vi "Disabled.vi"(7 "Robot Mode":T2, 10 "Match Info":T1={"Autonomous Elapsed Seconds"=0.0, "TeleOp Elapsed Seconds"=0.0, "Disabled Elapsed Seconds"=0.0, "Visited Autonomous"=FALSE, "Visited TeleOp"=FALSE, "Visited Disabled"=FALSE, "Autonomous Settings"={"Autonomous Style"=enum."Independent", "VI Refnum"=refnum}}, 11 "Call Context":T3) -> ()   [LabVIEW 2015]
doc: "This VI is called each time a disabled packet is received from the DS. It is often used to prepare for the next robot mode, to calibrate sensors, etc."
uses:
  <vilib>/Rock Robotics/WPI/DriverStation/WPI_DriverStationDerivedRobotMode.ctl
  <vilib>/Rock Robotics/WPI/DriverStation/WPI_DriverStationRobotMode2.ctl
  <vilib>/Rock Robotics/WPI/DriverStation/WPI_DriverStationMatch Info.ctl
  Robot Global Data.vi
panel:
  # "DISABLED.VI"
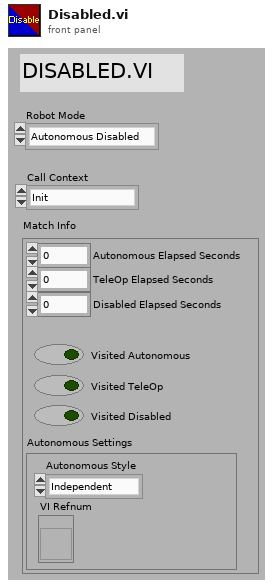
[diagram p1: front panel]
types:
  T1 = typedef "WPI_DriverStationMatch Info.ctl" = cluster{"Autonomous Elapsed Seconds":dbl, "TeleOp Elapsed Seconds":dbl, "Disabled Elapsed Seconds":dbl, "Visited Autonomous":bool, "Visited TeleOp":bool, "Visited Disabled":bool, "Autonomous Settings":cluster{"Autonomous Style":enum16{"Iterative", "Independent"}, "VI Refnum":refnum<vi>}}
  T2 = typedef "WPI_DriverStationRobotMode2.ctl" = enum16{"Autonomous Disabled", "Autonomous Enabled", "Teleop Disabled", "Teleop Enabled", "Disconnected", "Finish", "Test Disabled", "Test Enabled", "Emergency Stopped"}
  T3 = typedef "WPI_DriverStationDerivedRobotMode.ctl" = enum16{"Init", "Execute", "Stop"}
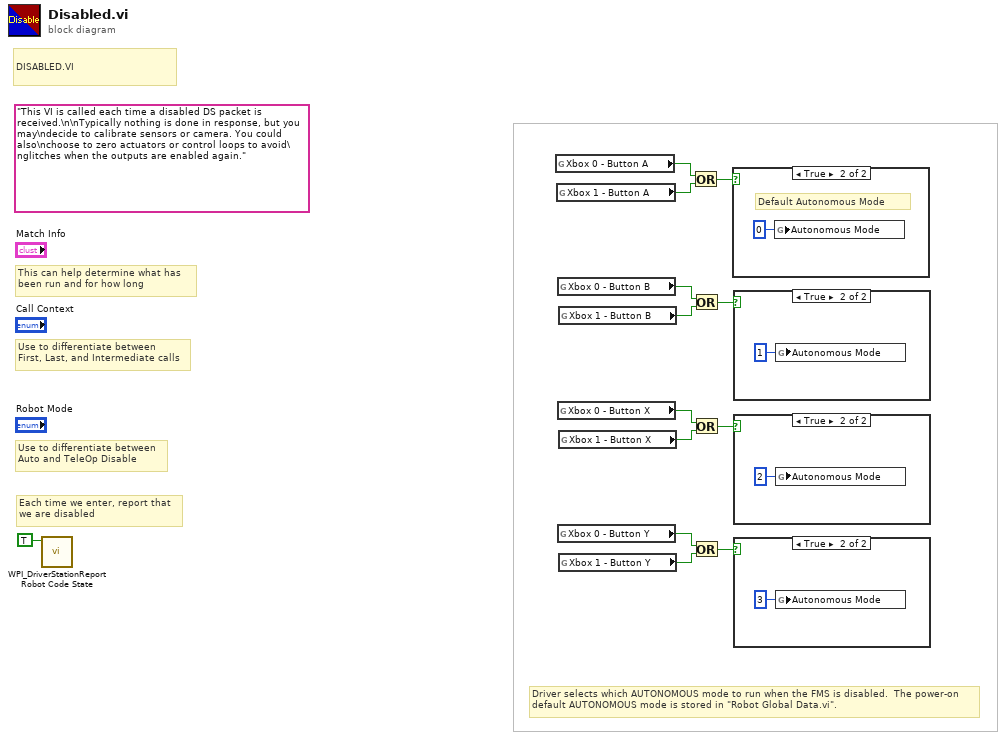
[diagram p0: block diagram]
diagram:
  (unwired) "This VI is called each time a disabled DS packet is received.\n\nTypically nothing is done in response, but you may\ndecide to calibrate sensors or camera. You could also\nchoose to zero actuators or control loops to avoid\nglitches when the outputs are enabled again."
  # "DISABLED.VI"
  # "Driver selects which AUTONOMOUS mode to run when the FMS is disabled.  The power-on default AUTONOMOUS mode is stored in \"Robot Global Data.vi\"."
  # "Each time we enter, report that\nwe are disabled"
  # "Use to differentiate between\nFirst, Last, and Intermediate calls"
  # "This can help determine what has\nbeen run and for how long"
  # "Use to differentiate between\nAuto and TeleOp Disable"
  n1 = call <vilib>:"WPI_DriverStationReport Robot Code State.vi"("Disabled"=TRUE ("Autonomous")) -> ()  [unwired: 10 in, 1 out]
  n2 = global read "Robot Global Data.vi" "Xbox 0 - Button A"() -> (w12:bool)
  n3 = global read "Robot Global Data.vi" "Xbox 1 - Button A"() -> (w11:bool)
  n4 = global read "Robot Global Data.vi" "Xbox 0 - Button B"() -> (w9:bool)
  n5 = global read "Robot Global Data.vi" "Xbox 0 - Button X"() -> (w6:bool)
  n6 = global read "Robot Global Data.vi" "Xbox 0 - Button Y"() -> (w3:bool)
  n7 = global read "Robot Global Data.vi" "Xbox 1 - Button B"() -> (w8:bool)
  n8 = global read "Robot Global Data.vi" "Xbox 1 - Button X"() -> (w5:bool)
  n9 = global read "Robot Global Data.vi" "Xbox 1 - Button Y"() -> (w2:bool)
  n10 = Or(x=w12, y=w11) -> (x .or. y?=w10:bool)
  n11 = Or(x=w9, y=w8) -> (x .or. y?=w7:bool)
  n12 = Or(x=w6, y=w5) -> (x .or. y?=w4:bool)
  n13 = Or(x=w3, y=w2) -> (x .or. y?=w1:bool)
  n14 = case shown="True" w10 {
    frame False {
    }
    frame True {
      # "Default Autonomous Mode"
      n15 = global write "Robot Global Data.vi" "Autonomous Mode"(i8 0 ("Autonomous Mode")) -> ()
    }
  }
  n16 = case shown="True" w7 {
    frame False {
    }
    frame True {
      n17 = global write "Robot Global Data.vi" "Autonomous Mode"(i8 1 ("Autonomous Mode")) -> ()
    }
  }
  n18 = case shown="True" w4 {
    frame False {
    }
    frame True {
      n19 = global write "Robot Global Data.vi" "Autonomous Mode"(i8 2 ("Autonomous Mode")) -> ()
    }
  }
  n20 = case shown="True" w1 {
    frame False {
    }
    frame True {
      n21 = global write "Robot Global Data.vi" "Autonomous Mode"(i8 3 ("Autonomous Mode")) -> ()
    }
  }
